vi "BuildConfigsFromFrontPanel.vi"(10 "AllControlsRefs":T25, 11 "InstruConfig":T1={"Mode"="", "InstrumentMode"={"MainDAQ_Selector"=enum."None", "LaserCtrlMethod"=enum."SRS_DG535", "InstruMode"=enum."fsLDPI"}, "CommuniationSettings"={"SDG_II"="", "DG535"="", "BNC565"="", "EPM2000"="", "NI-DAQmx"="", "Micos"={"Simulation"=FALSE, "ComPort"="", "Serial Config"={"Baud Rate"=0, "Parity"=0, "Data Bits"=0, "Stop Bits"=0, "Flow Control"=0}, "#Axis"=0}, "ESP300"={"Simulation"=FALSE, "ComPort"="", "Serial Config"={"Baud Rate"=0, "Parity"=0, "Data Bits"=0, "Stop Bits"=0, "Flow Control"=0}, "#Axis"=0}}, "DG535"={"Trigger"={"Trigger Mode"=enum."Internal", "Internal/Burst Rate"=0.0, "External  Level"=0.0, "Impedance"=FALSE, "Slope"=FALSE}, "Delays"=[], "Output"=[]}, "Gage_Config"={"Acquisition"={"Sample Rate"=0.0, "Mode"=0, "Start (0)"=0.0, "Depth"=0.0, "Segment Size"=0.0, "Trigger Delay"=0.0, "Trigger Timeout"=0.0, "Trigger Holdoff"=0.0, "Clock mode"=enum."Internal", "Segment"=1}, "Channels"=[], "Trigger"={"Slope"=0, "Level"=0, "Source"=0, "External Range"=0, "External Coupling"=0, "External"=FALSE, "Disable"=FALSE, "External Impedance"=0}, "Mode(Gage)"=enum."Normal"}, "AnalogDisc_Config"={"Acqusition"={"Freq(Hz,SampleRate)"=0.0, "BufferSize"=0, "Mode"=enum."Single", "RecordLength(s)"=0.0}, "Channels"=[], "Trigger"={"TriggerSource"=enum."None", "Timeout(s)"=0.0, "Holdoff(s)"=0.0, "Position/Delay(s)"=0.0}, "AnalogTrigger"={"Channel"=0, "Polarity"=enum."Rising", "Type"=enum."Edge", "Level(V)"=0.0, "Filter"=enum."Decimate", "Hysterisis(V)"=0.0}}, "Micos"={"Velocity"=0.0, "Acceleration"=0.0}, "ESP300"={"Velocity"=[], "Acceleration"=[]}, "EPM2000"={"Factor(A)"=0.0, "Factor(B)"=0.0}, "ProcessMethod"={"TopLine"=0.0, "Threshold"=0.0, "Baseline"=0.0, "ZeroOffset"=0.0, "Processing Mode"=enum."None"}, "Timing(LDPI)"={"Delay(PI)"=0.0, "Delay(Rejection)"=0.0, "NoDelayOffset"=0.0, "RepRate(Hz)"=0.0}, "Cali."=[0.0707, 0.16163, 0.02539], "BNC_Config"={"System"={"Rep.Rate"=1000.0, "Sys Ext Mode"=enum."Triggered", "Mode"=enum."Single Shot"}, "Channels"=[]}} {"Cali." format="%#.6f"; "Timing(LDPI)"."Delay(PI)" format="%#_6p"; "Timing(LDPI)"."Delay(Rejection)" format="%#_6p"; "Timing(LDPI)"."NoDelayOffset" format="%#_6p"; "DG535"."Trigger"."External  Level" min=-2.56 max=2.56 format="%.2f"; "DG535"."Trigger"."Internal/Burst Rate" min=0.001 max=1000000.0 format="%.3f"; "DG535"."Delays"."Delay" format="%#_6p"; "DG535"."Output"."Offset" min=-3.0 max=4.0 format="%.2f"; "DG535"."Output"."Amplitude" min=-3.0 max=4.0 format="%.2f"; "ProcessMethod"."Threshold" format="%#_6p"; "Gage_Config"."Trigger"."External Impedance" items=["50 Ohm", "HiZ"]; "Gage_Config"."Trigger"."External Coupling" items=["DC", "AC"]; "Gage_Config"."Trigger"."External Range" min=2000 max=10000 step=8000; "Gage_Config"."Trigger"."Slope" items=["Rising", "Falling"]; "Gage_Config"."Trigger"."Level" min=-100 max=100; "Gage_Config"."Trigger"."Source" min=0 max=64 step=1; "Gage_Config"."Channels"."Impedance" min=50 max=1000000 step=999950; "Gage_Config"."Channels"."Coupling" items=["DC", "AC"]; "Gage_Config"."Acquisition"."Segment Size" min=256.0 step=128.0; "Gage_Config"."Acquisition"."Trigger Delay" min=0.0 step=128.0; "Gage_Config"."Acquisition"."Trigger Timeout" format="%.0p"; "Gage_Config"."Acquisition"."Trigger Holdoff" min=0.0 step=128.0; "Gage_Config"."Acquisition"."Depth" min=256.0 step=128.0; "Gage_Config"."Acquisition"."Mode" items=["Single", "Dual", "Quad", "Octal"]; "Gage_Config"."Acquisition"."Sample Rate" format="%.0p"; "AnalogDisc_Config"."AnalogTrigger"."Level(V)" format="%#_6p"; "AnalogDisc_Config"."AnalogTrigger"."Hysterisis(V)" format="%#_6p"; "AnalogDisc_Config"."Acqusition"."RecordLength(s)" format="%#_6p"; "AnalogDisc_Config"."Acqusition"."Freq(Hz,SampleRate)" format="%#_6p"; "AnalogDisc_Config"."Trigger"."Position/Delay(s)" format="%#_6p"; "AnalogDisc_Config"."Trigger"."Holdoff(s)" format="%#_6p"; "AnalogDisc_Config"."Trigger"."Timeout(s)" format="%#_6p"}) -> (2 "InstruConfig out":T1={"Mode"="", "InstrumentMode"={"MainDAQ_Selector"=enum."None", "LaserCtrlMethod"=enum."SRS_DG535", "InstruMode"=enum."fsLDPI"}, "CommuniationSettings"={"SDG_II"="", "DG535"="", "BNC565"="", "EPM2000"="", "NI-DAQmx"="", "Micos"={"Simulation"=FALSE, "ComPort"="", "Serial Config"={"Baud Rate"=0, "Parity"=0, "Data Bits"=0, "Stop Bits"=0, "Flow Control"=0}, "#Axis"=0}, "ESP300"={"Simulation"=FALSE, "ComPort"="", "Serial Config"={"Baud Rate"=0, "Parity"=0, "Data Bits"=0, "Stop Bits"=0, "Flow Control"=0}, "#Axis"=0}}, "DG535"={"Trigger"={"Trigger Mode"=enum."Internal", "Internal/Burst Rate"=0.0, "External  Level"=0.0, "Impedance"=FALSE, "Slope"=FALSE}, "Delays"=[], "Output"=[]}, "Gage_Config"={"Acquisition"={"Sample Rate"=0.0, "Mode"=0, "Start (0)"=0.0, "Depth"=0.0, "Segment Size"=0.0, "Trigger Delay"=0.0, "Trigger Timeout"=0.0, "Trigger Holdoff"=0.0, "Clock mode"=enum."Internal", "Segment"=1}, "Channels"=[], "Trigger"={"Slope"=0, "Level"=0, "Source"=0, "External Range"=0, "External Coupling"=0, "External"=FALSE, "Disable"=FALSE, "External Impedance"=0}, "Mode(Gage)"=enum."Normal"}, "AnalogDisc_Config"={"Acqusition"={"Freq(Hz,SampleRate)"=0.0, "BufferSize"=0, "Mode"=enum."Single", "RecordLength(s)"=0.0}, "Channels"=[], "Trigger"={"TriggerSource"=enum."None", "Timeout(s)"=0.0, "Holdoff(s)"=0.0, "Position/Delay(s)"=0.0}, "AnalogTrigger"={"Channel"=0, "Polarity"=enum."Rising", "Type"=enum."Edge", "Level(V)"=0.0, "Filter"=enum."Decimate", "Hysterisis(V)"=0.0}}, "Micos"={"Velocity"=0.0, "Acceleration"=0.0}, "ESP300"={"Velocity"=[], "Acceleration"=[]}, "EPM2000"={"Factor(A)"=0.0, "Factor(B)"=0.0}, "ProcessMethod"={"TopLine"=0.0, "Threshold"=0.0, "Baseline"=0.0, "ZeroOffset"=0.0, "Processing Mode"=enum."None"}, "Timing(LDPI)"={"Delay(PI)"=0.0, "Delay(Rejection)"=0.0, "NoDelayOffset"=0.0, "RepRate(Hz)"=0.0}, "Cali."=[0.0707, 0.16163, 0.02539], "BNC_Config"={"System"={"Rep.Rate"=1000.0, "Sys Ext Mode"=enum."Triggered", "Mode"=enum."Single Shot"}, "Channels"=[]}} {"Cali." format="%#.6f"; "Timing(LDPI)"."Delay(PI)" format="%#_6p"; "Timing(LDPI)"."Delay(Rejection)" format="%#_6p"; "Timing(LDPI)"."NoDelayOffset" format="%#_6p"; "DG535"."Trigger"."External  Level" min=-2.56 max=2.56 format="%.2f"; "DG535"."Trigger"."Internal/Burst Rate" min=0.001 max=1000000.0 format="%.3f"; "DG535"."Delays"."Delay" format="%#_6p"; "DG535"."Output"."Offset" min=-3.0 max=4.0 format="%.2f"; "DG535"."Output"."Amplitude" min=-3.0 max=4.0 format="%.2f"; "ProcessMethod"."Threshold" format="%#_6p"; "Gage_Config"."Trigger"."External Impedance" items=["50 Ohm", "HiZ"]; "Gage_Config"."Trigger"."External Coupling" items=["DC", "AC"]; "Gage_Config"."Trigger"."External Range" min=2000 max=10000 step=8000; "Gage_Config"."Trigger"."Slope" items=["Rising", "Falling"]; "Gage_Config"."Trigger"."Level" min=-100 max=100; "Gage_Config"."Trigger"."Source" min=0 max=64 step=1; "Gage_Config"."Channels"."Impedance" min=50 max=1000000 step=999950; "Gage_Config"."Channels"."Coupling" items=["DC", "AC"]; "Gage_Config"."Acquisition"."Segment Size" min=256.0 step=128.0; "Gage_Config"."Acquisition"."Trigger Delay" min=0.0 step=128.0; "Gage_Config"."Acquisition"."Trigger Timeout" format="%.0p"; "Gage_Config"."Acquisition"."Trigger Holdoff" min=0.0 step=128.0; "Gage_Config"."Acquisition"."Depth" min=256.0 step=128.0; "Gage_Config"."Acquisition"."Mode" items=["Single", "Dual", "Quad", "Octal"]; "Gage_Config"."Acquisition"."Sample Rate" format="%.0p"; "AnalogDisc_Config"."AnalogTrigger"."Level(V)" format="%#_6p"; "AnalogDisc_Config"."AnalogTrigger"."Hysterisis(V)" format="%#_6p"; "AnalogDisc_Config"."Acqusition"."RecordLength(s)" format="%#_6p"; "AnalogDisc_Config"."Acqusition"."Freq(Hz,SampleRate)" format="%#_6p"; "AnalogDisc_Config"."Trigger"."Position/Delay(s)" format="%#_6p"; "AnalogDisc_Config"."Trigger"."Holdoff(s)" format="%#_6p"; "AnalogDisc_Config"."Trigger"."Timeout(s)" format="%#_6p"})   [LabVIEW 2013]
uses:
  ControlDef/InstrumentConfiguration.ctl
  ControlDef/MainDAQ_Selector.ctl
  ControlDef/LaserCtrl_Method.ctl
  ControlDef/InstruMode_Typedef.ctl
  <instrlib>/DG535/Command/Set Trigger.ctl
  <instrlib>/DG535/Command/DG535_TriggerMode.ctl
  <instrlib>/DG535/Command/Set Delay.ctl
  <instrlib>/DG535/Command/DG535_Channel.ctl
  <instrlib>/DG535/Command/Set Output.ctl
  <instrlib>/DG535/Command/DG535_Output.ctl
  <instrlib>/GageLv_uic/VI/Gage_Configs.ctl
  <instrlib>/AnalogDiscSDKLv/VIs/DWF_AnalogIn_Configurations.ctl
  <instrlib>/AnalogDiscSDKLv/VIs/DWF_AcqMode.ctl
  <instrlib>/AnalogDiscSDKLv/VIs/DWF_Filter.ctl
  <instrlib>/AnalogDiscSDKLv/VIs/DWF_TrigSrc.ctl
  <instrlib>/AnalogDiscSDKLv/VIs/DWF_TrigCond.ctl
  <instrlib>/AnalogDiscSDKLv/VIs/DWF_TrigType.ctl
  ControlDef/ProcessingMode.ctl
  Hardware/BNC(QuantumComposers)/BNC_Configs.ctl
  ControlDef/InstrumentSpecificControls/UIC-AToF/InitializationParams_BNC565_2Ch_AToF.ctl
  Hardware/BNC(QuantumComposers)/Command/Set C-Input.ctl
  Hardware/BNC(QuantumComposers)/Command/Set C-Mode.ctl
  Hardware/BNC(QuantumComposers)/Command/Set C-Output.ctl
  Hardware/BNC(QuantumComposers)/Command/Set C-Enable.ctl
  ControlDef/AllControlsRefs.ctl
  <instrlib>/DG535/SRS_DG535_Lib.lvlib
  <instrlib>/GageLv_uic/Gage.lvlib
  <instrlib>/AnalogDiscSDKLv/AnalogDiscSDKLv.lvlib
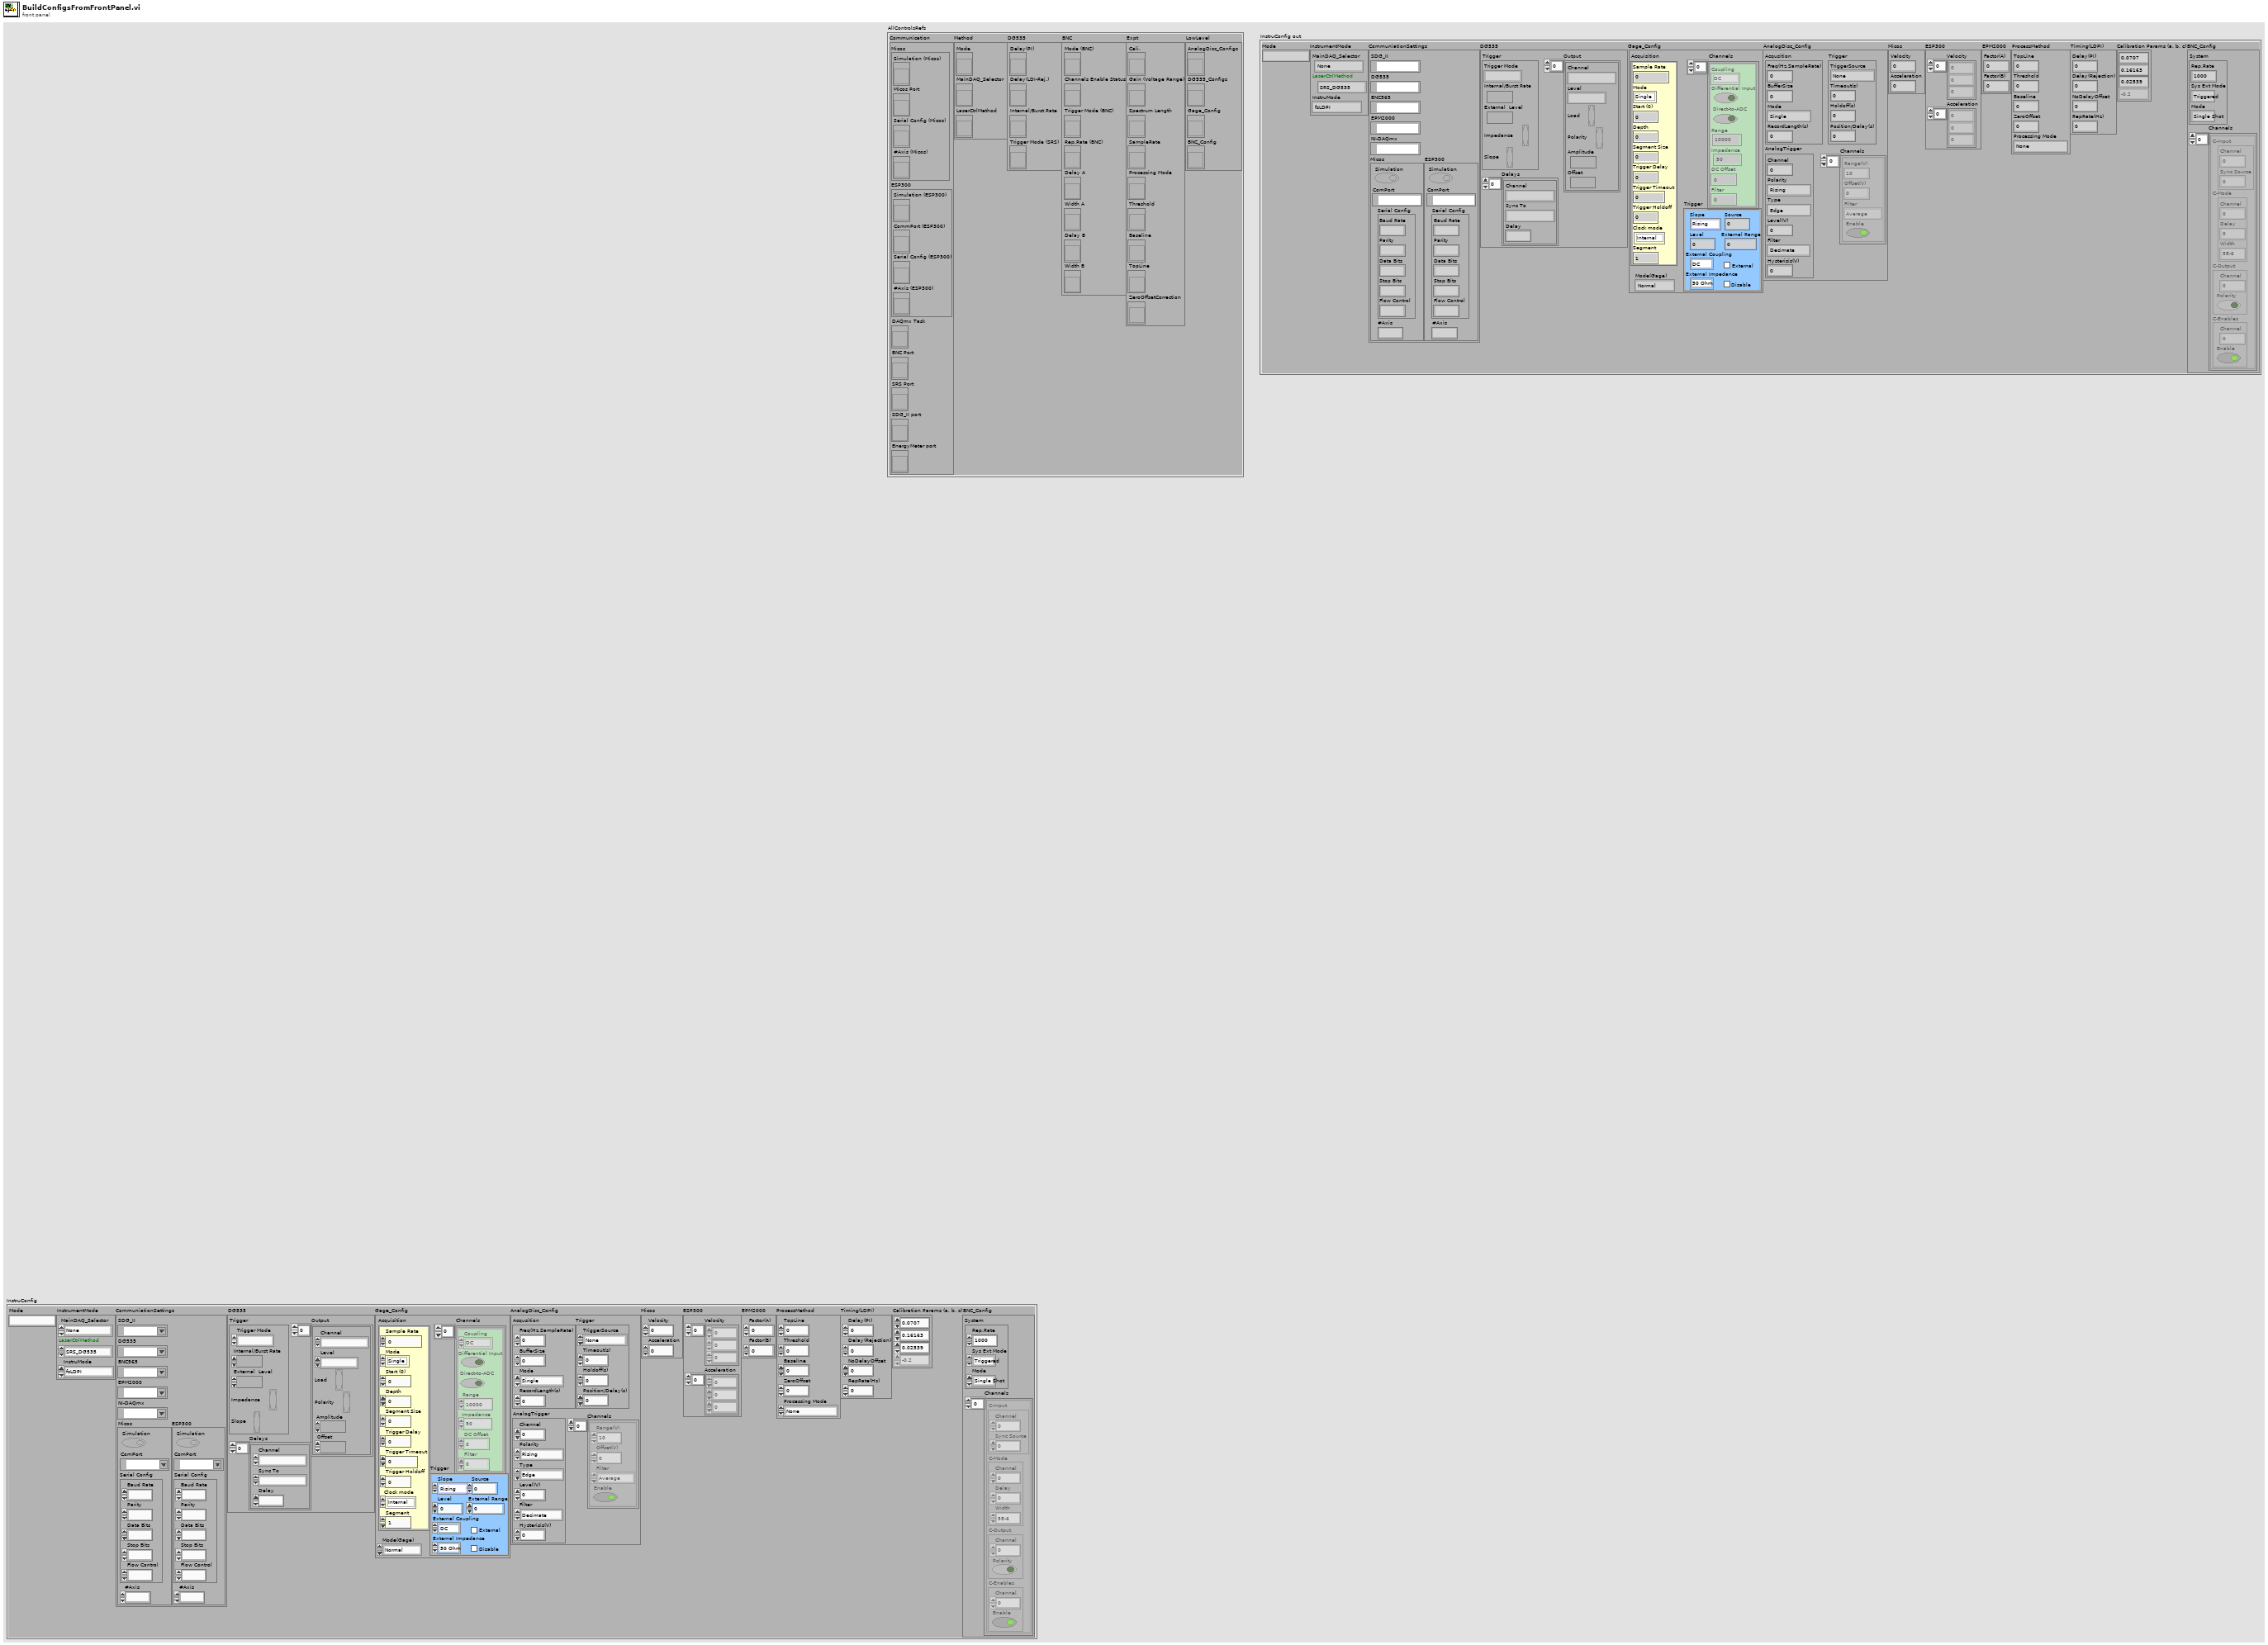
[diagram p1: front panel]
types:
  T1 = typedef "InstrumentConfiguration.ctl" = cluster{"Mode":string, "InstrumentMode":cluster{"MainDAQ_Selector":T2, "LaserCtrlMethod":T3, "InstruMode":T4}, "CommuniationSettings":cluster{"SDG_II":refnum<visa-resource-name>, "DG535":refnum<visa-resource-name>, "BNC565":refnum<visa-resource-name>, "EPM2000":refnum<visa-resource-name>, "NI-DAQmx":refnum<visa-resource-name>, "Micos":cluster{"Simulation":bool, "ComPort":refnum<visa-resource-name>, "Serial Config":cluster{"Baud Rate":u32, "Parity":u16, "Data Bits":u16, "Stop Bits":u16, "Flow Control":u16}, "#Axis":i32}, "ESP300":cluster{"Simulation":bool, "ComPort":refnum<visa-resource-name>, "Serial Config":cluster{"Baud Rate":u32, "Parity":u16, "Data Bits":u16, "Stop Bits":u16, "Flow Control":u16}, "#Axis":i32}}, "DG535":cluster{"Trigger":T5, "Delays":T7[], "Output":T9[]}, "Gage_Config":T11, "AnalogDisc_Config":T12, "Micos":cluster{"Velocity":dbl, "Acceleration":dbl}, "ESP300":cluster{"Velocity":dbl[], "Acceleration":dbl[]}, "EPM2000":cluster{"Factor(A)":dbl, "Factor(B)":dbl}, "ProcessMethod":cluster{"TopLine":dbl, "Threshold":dbl, "Baseline":dbl, "ZeroOffset":dbl, "Processing Mode":T18}, "Timing(LDPI)":cluster{"Delay(PI)":dbl, "Delay(Rejection)":dbl, "NoDelayOffset":dbl, "RepRate(Hz)":dbl}, "Cali.":dbl[], "BNC_Config":T19}
  T2 = typedef "MainDAQ_Selector.ctl" = enum16{"None", "Gage", "Gage_AdvMultiRec_8bit1Ch", "IonWerks_TDCx4", "Tektronics", "KnifeEdge_Emu", "AnalogDisc", "Gage_AMR_8bit2Ch", "Gage_AMR_16bit1Ch", "Gage_AMR_16bit2Ch"}
  T3 = typedef "LaserCtrl_Method.ctl" = enum16{"SRS_DG535", "BNC", "SDG_II"}
  T4 = typedef "InstruMode_Typedef.ctl" = enum16{"fsLDPI", "nsLDPI", "nsLD-fsPI", "GenericTOF", "BeamProfiling"}
  T5 = typedef "SRS_DG535_Lib.lvlib/Set Trigger.ctl" = cluster{"Trigger Mode":T6, "Internal/Burst Rate":dbl, "External  Level":sgl, "Impedance":bool, "Slope":bool}
  T6 = typedef "SRS_DG535_Lib.lvlib/DG535_TriggerMode.ctl" = enum16{"Internal", "External", "SingleShot", "Burst", "Line"}
  T7 = typedef "SRS_DG535_Lib.lvlib/Set Delay.ctl" = cluster{"Channel":T8, "Sync To":T8, "Delay":dbl}
  T8 = typedef "SRS_DG535_Lib.lvlib/DG535_Channel.ctl" = enum16{"Trigger Input", "T0 Output", "A Output", "B Output", "AB Output", "C Output", "D Output", "CD Output", "NULL"}
  T9 = typedef "SRS_DG535_Lib.lvlib/Set Output.ctl" = cluster{"Channel":T8, "Level":T10, "Load":bool, "Polarity":bool, "Amplitude":dbl, "Offset":dbl}
  T10 = typedef "SRS_DG535_Lib.lvlib/DG535_Output.ctl" = enum16{"TTL", "NIM", "ECL", "Variable"}
  T11 = typedef "Gage.lvlib/Gage_Configs.ctl" = cluster{"Acquisition":cluster{"Sample Rate":dbl, "Mode":u16, "Start (0)":dbl, "Depth":dbl, "Segment Size":dbl, "Trigger Delay":dbl, "Trigger Timeout":dbl, "Trigger Holdoff":dbl, "Clock mode":enum16{"Internal", "External", "Reference"}, "Segment":u32}, "Channels":cluster{"Coupling":u16, "Differential Input":bool, "Direct-to-ADC":bool, "Range":u32, "Impedance":u32, "DC Offset":i32, "Filter":i32}[], "Trigger":cluster{"Slope":u16, "Level":i32, "Source":i32, "External Range":u32, "External Coupling":u16, "External":bool, "Disable":bool, "External Impedance":u16}, "Mode(Gage)":enum16{"Normal", "Continuous", "MultiRecord", "HwAverage"}}
  T12 = typedef "AnalogDiscSDKLv.lvlib/DWF_AnalogIn_Configurations.ctl" = cluster{"Acqusition":cluster{"Freq(Hz,SampleRate)":dbl, "BufferSize":i32, "Mode":T13, "RecordLength(s)":dbl}, "Channels":cluster{"Range(V)":dbl, "Offset(V)":dbl, "Filter":T14, "Enable":bool}[], "Trigger":cluster{"TriggerSource":T15, "Timeout(s)":dbl, "Holdoff(s)":dbl, "Position/Delay(s)":dbl}, "AnalogTrigger":cluster{"Channel":i32, "Polarity":T16, "Type":T17, "Level(V)":dbl, "Filter":T14, "Hysterisis(V)":dbl}}
  T13 = typedef "AnalogDiscSDKLv.lvlib/DWF_AcqMode.ctl" = enum16{"Single", "ScanShift", "ScanScreen", "Record"}
  T14 = typedef "AnalogDiscSDKLv.lvlib/DWF_Filter.ctl" = enum16{"Decimate", "Average", "MinMax"}
  T15 = typedef "AnalogDiscSDKLv.lvlib/DWF_TrigSrc.ctl" = enum16{"None", "PC", "DetectorAnalogIn", "DetectorDigitalIn", "AnalogIn", "DigitalIn", "DigitalOut", "AnalogOut1", "AnalogOut2", "AnalogOut3", "AnalogOut4", "External1", "External2", "External3", "External4"}
  T16 = typedef "AnalogDiscSDKLv.lvlib/DWF_TrigCond.ctl" = enum16{"Rising", "Falling"}
  T17 = typedef "AnalogDiscSDKLv.lvlib/DWF_TrigType.ctl" = enum16{"Edge", "Pulse", "Transition"}
  T18 = typedef "ProcessingMode.ctl" = enum16{"None", "Drop by Threshold", "TDC Simulate", "SetFilter"}
  T19 = typedef "BNC_Configs.ctl" = cluster{"System":cluster{"Rep.Rate":dbl, "Sys Ext Mode":enum16{"Disabled", "Triggered", "Gated", "Triggered & Gated"}, "Mode":enum16{"Normal", "Single Shot", "Duty Cycle", "Burst"}}, "Channels":T20[]}
  T20 = typedef "InitializationParams_BNC565_2Ch_AToF.ctl" = cluster{"C-Input":T21, "C-Mode":T22, "C-Output":T23, "C-Enables":T24}
  T21 = typedef "Set C-Input.ctl" = cluster{"Channel":i32, "Sync Source":i32}
  T22 = typedef "Set C-Mode.ctl" = cluster{"Channel":i32, "Delay":dbl, "Width":dbl}
  T23 = typedef "Set C-Output.ctl" = cluster{"Channel":i32, "Polarity":bool}
  T24 = typedef "Set C-Enable.ctl" = cluster{"Channel":i32, "Enable":bool}
  T25 = typedef "AllControlsRefs.ctl" = cluster{"Communication":cluster{"Micos":cluster{"Simulation (Micos)":refnum<vi>, "Micos Port":refnum<vi>, "Serial Config (Micos)":refnum<vi>, "#Axis (Micos)":refnum<vi>}, "ESP300":cluster{"Simulation (ESP300)":refnum<vi>, "CommPort (ESP300)":refnum<vi>, "Serial Config (ESP300)":refnum<vi>, "#Axis (ESP300)":refnum<vi>}, "DAQmx Task":refnum<vi>, "BNC Port":refnum<vi>, "SRS Port":refnum<vi>, "SDG_II port":refnum<vi>, "EnergyMeter port":refnum<vi>}, "Method":cluster{"Mode":refnum<vi>, "MainDAQ_Selector":refnum<vi>, "LaserCtrlMethod":refnum<vi>}, "DG535":cluster{"Delay(PI)":refnum<vi>, "Delay(LDI-Rej.)":refnum<vi>, "Internal/Burst Rate":refnum<vi>, "Trigger Mode (SRS)":refnum<vi>}, "BNC":cluster{"Mode (BNC)":refnum<vi>, "Channels Enable Status":refnum<vi>, "Trigger Mode (BNC)":refnum<vi>, "Rep.Rate (BNC)":refnum<vi>, "Delay A":refnum<vi>, "Width A":refnum<vi>, "Delay B":refnum<vi>, "Width B":refnum<vi>}, "Expt":cluster{"Cali.":refnum<vi>, "Gain (Voltage Range)":refnum<vi>, "Spectrum Length":refnum<vi>, "SampleRate":refnum<vi>, "Processing Mode":refnum<vi>, "Threshold":refnum<vi>, "Baseline":refnum<vi>, "TopLine":refnum<vi>, "ZeroOffsetCorrection":refnum<vi>}, "LowLevel":cluster{"AnalogDisc_Configs":refnum<vi>, "DG535_Configs":refnum<vi>, "Gage_Config":refnum<vi>, "BNC_Config":refnum<vi>}}
  T26 = cluster{"Trigger":T5, "Delays":T7[], "Output":T9[]}
  T27 = cluster{"Baud Rate":u32, "Parity":u16, "Data Bits":u16, "Stop Bits":u16, "Flow Control":u16}
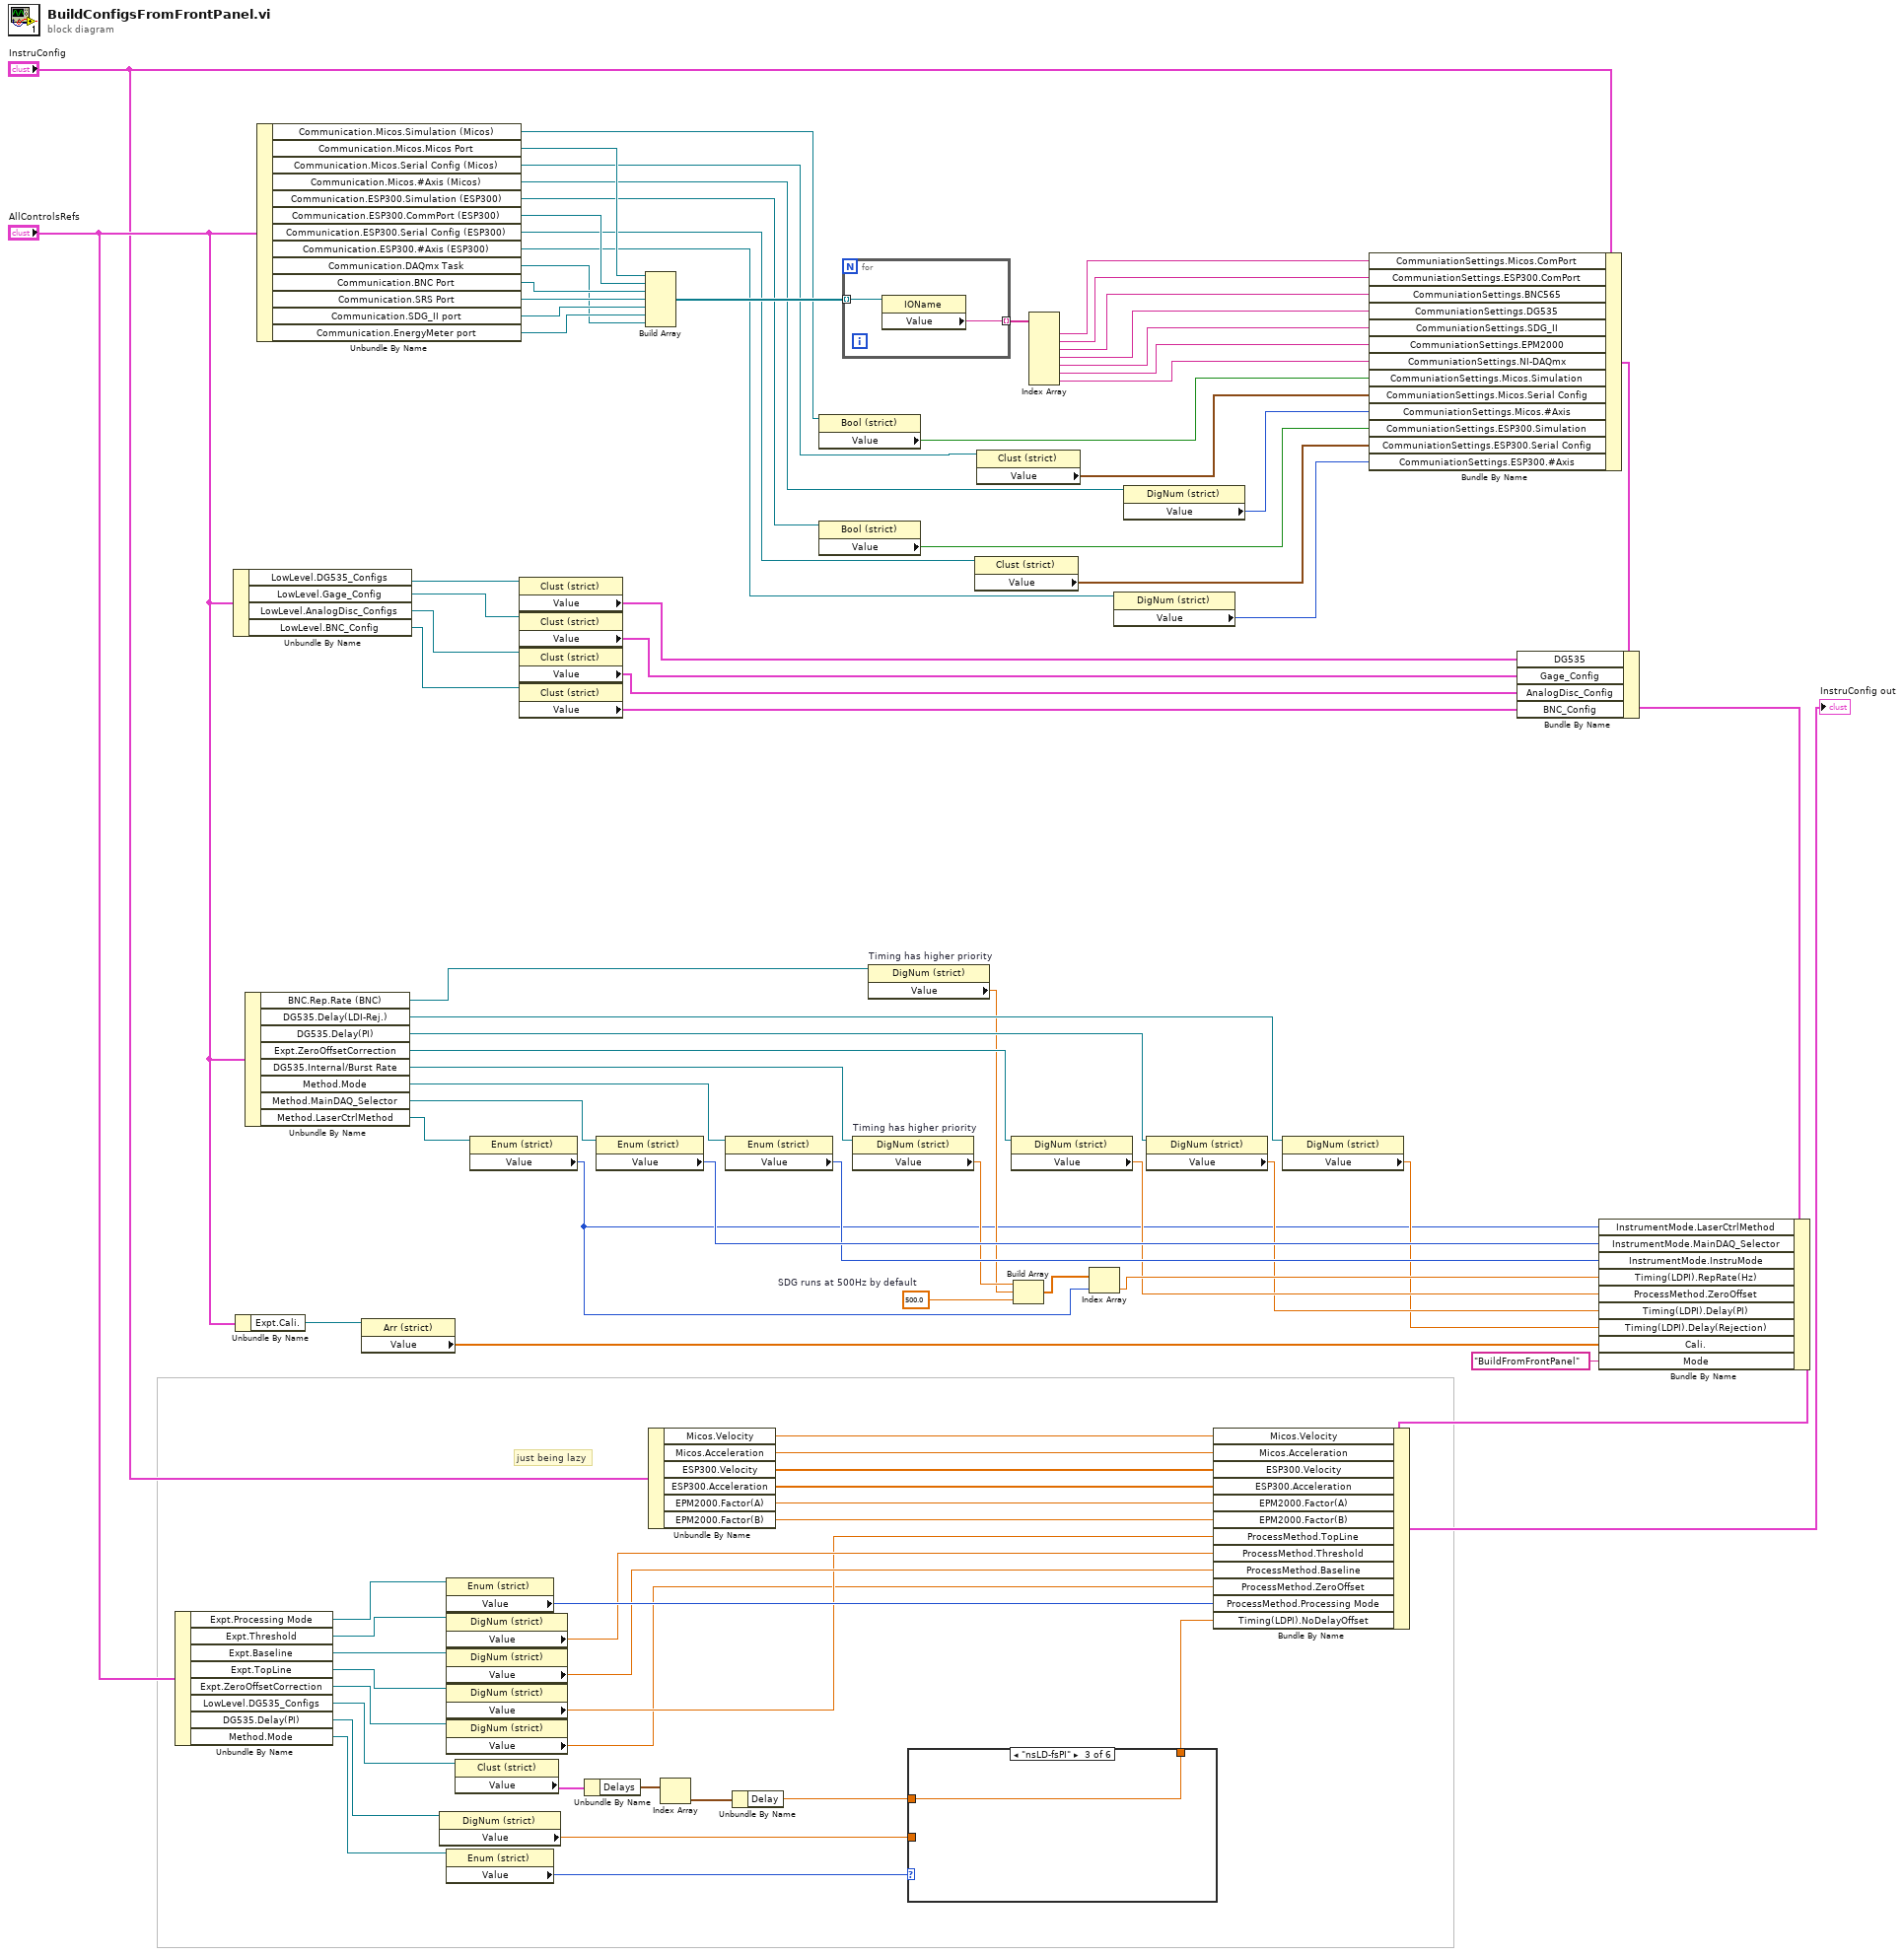
[diagram p0: block diagram]
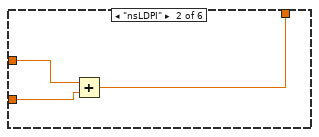
[diagram p3: hidden frame]
diagram:
  w34 = 500.0  # SDG runs at 500Hz by default
  # "just being lazy"
  n1 = Unbundle By Name("AllControlsRefs") -> ("Expt.Processing Mode"=w28:refnum<vi>, "Expt.Threshold"=w27:refnum<vi>, "Expt.Baseline"=w26:refnum<vi>, "Expt.TopLine"=w25:refnum<vi>, "Expt.ZeroOffsetCorrection"=w24:refnum<vi>, "LowLevel.DG535_Configs"=w10:refnum<vi>, "DG535.Delay(PI)"=w2:refnum<vi>, "Method.Mode"=w6:refnum<vi>)
  n2 = Unbundle By Name("AllControlsRefs") -> ("LowLevel.DG535_Configs"=w83:refnum<vi>, "LowLevel.Gage_Config"=w82:refnum<vi>, "LowLevel.AnalogDisc_Configs"=w81:refnum<vi>, "LowLevel.BNC_Config"=w65:refnum<vi>)
  n3 = Unbundle By Name("AllControlsRefs") -> ("Expt.Cali."=w66:refnum<vi>)
  n4 = Unbundle By Name("AllControlsRefs") -> ("BNC.Rep.Rate (BNC)"=w35:refnum<vi>, "DG535.Delay(LDI-Rej.)"=w67:refnum<vi>, "DG535.Delay(PI)"=w68:refnum<vi>, "Expt.ZeroOffsetCorrection"=w69:refnum<vi>, "DG535.Internal/Burst Rate"=w70:refnum<vi>, "Method.Mode"=w73:refnum<vi>, "Method.MainDAQ_Selector"=w72:refnum<vi>, "Method.LaserCtrlMethod"=w71:refnum<vi>)
  n5 = Unbundle By Name("AllControlsRefs") -> ("Communication.Micos.Simulation (Micos)"=w80:refnum<vi>, "Communication.Micos.Micos Port"=w90:refnum<vi>, "Communication.Micos.Serial Config (Micos)"=w78:refnum<vi>, "Communication.Micos.#Axis (Micos)"=w77:refnum<vi>, "Communication.ESP300.Simulation (ESP300)"=w79:refnum<vi>, "Communication.ESP300.CommPort (ESP300)"=w89:refnum<vi>, "Communication.ESP300.Serial Config (ESP300)"=w76:refnum<vi>, "Communication.ESP300.#Axis (ESP300)"=w75:refnum<vi>, "Communication.DAQmx Task"=w74:refnum<vi>, "Communication.BNC Port"=w88:refnum<vi>, "Communication.SRS Port"=w87:refnum<vi>, "Communication.SDG_II port"=w86:refnum<vi>, "Communication.EnergyMeter port"=w85:refnum<vi>)
  n6 = property class="Arr (strict)"(reference=w66) -> ("Value"=w42:dbl[])  [unwired: 1 in, 2 out]
  n7 = property class="DigNum (strict)"(reference=w2) -> ("Value"=w1:dbl)  [unwired: 1 in, 2 out]
  n8 = property class="Enum (strict)"(reference=w28) -> ("Value"=w23:T18)  [unwired: 1 in, 2 out]
  n9 = property class="DigNum (strict)"(reference=w27) -> ("Value"=w22:dbl)  [unwired: 1 in, 2 out]
  n10 = property class="DigNum (strict)"(reference=w26) -> ("Value"=w21:dbl)  [unwired: 1 in, 2 out]
  n11 = property class="DigNum (strict)"(reference=w25) -> ("Value"=w20:dbl)  [unwired: 1 in, 2 out]
  n12 = property class="DigNum (strict)"(reference=w24) -> ("Value"=w19:dbl)  [unwired: 1 in, 2 out]
  n13 = property class="Enum (strict)"(reference=w6) -> ("Value"=w5:T4)  [unwired: 1 in, 2 out]
  n14 = property class="Clust (strict)"(reference=w10) -> ("Value"=w9:T26)  [unwired: 1 in, 2 out]
  n15 = property class="Enum (strict)"(reference=w71) -> ("Value"=w30:T3)  [unwired: 1 in, 2 out]
  n16 = property class="Clust (strict)"(reference=w83) -> ("Value"=w62:T26)  [unwired: 1 in, 2 out]
  n17 = property class="Clust (strict)"(reference=w82) -> ("Value"=w61:T11)  [unwired: 1 in, 2 out]
  n18 = property class="Clust (strict)"(reference=w81) -> ("Value"=w60:T12)  [unwired: 1 in, 2 out]
  n19 = property class="Clust (strict)"(reference=w65) -> ("Value"=w59:T19)  [unwired: 1 in, 2 out]
  n20 = Unbundle By Name(w9) -> ("Delays"=w8:T7[])
  n21 = property class="Enum (strict)"(reference=w72) -> ("Value"=w41:T2)  [unwired: 1 in, 2 out]
  n22 = Build Array(w90, w89, w88, w87, w86, w85, w74) -> (w84:refnum<vi>[])
  n23 = Unbundle By Name("InstruConfig") -> ("Micos.Velocity"=w17:dbl, "Micos.Acceleration"=w16:dbl, "ESP300.Velocity"=w15:dbl[], "ESP300.Acceleration"=w14:dbl[], "EPM2000.Factor(A)"=w13:dbl, "EPM2000.Factor(B)"=w12:dbl)
  n24 = Index Array(array=w8) -> (element=w7:T7)  [unwired: 1 in]
  n25 = property class="Enum (strict)"(reference=w73) -> ("Value"=w40:T4)  [unwired: 1 in, 2 out]
  n26 = Unbundle By Name(w7) -> ("Delay"=w3:dbl)
  n27 = property class="Bool (strict)"(reference=w80) -> ("Value"=w49:bool)  [unwired: 1 in, 2 out]
  n28 = property class="Bool (strict)"(reference=w79) -> ("Value"=w46:bool)  [unwired: 1 in, 2 out]
  n29 = for {
    tunnel: w84 -> [w92] mode=indexing
    tunnel: [w91] -> w57 mode=indexing
    n30 = property class="IOName"(reference=w92) -> ("Value"=w91:string)  [unwired: 1 in, 2 out]
  }
  n31 = property on="Timing has higher priority" class="DigNum (strict)"(reference=w70) -> ("Value"=w33:dbl)  [unwired: 1 in, 2 out]
  n32 = property on="Timing has higher priority" class="DigNum (strict)"(reference=w35) -> ("Value"=w32:dbl)  [unwired: 1 in, 2 out]
  n33 = case shown="\"nsLD-fsPI\"" w5 {
    tunnel: [w93 w94 w97 _ _ _] -> w4
    tunnel: w3 -> [w93 w95 w97 _ _ _]
    tunnel: w1 -> [_ w96 _ _ _ _]
    frame "fsLDPI" {
    }
    frame "nsLDPI" {
      n34 = Add(x=w95, y=w96) -> (x+y=w94:dbl)
    }
    frame "nsLD-fsPI" {
    }
    frame "GenericTOF" {
    }
    frame Default {
    }
    frame "BeamProfiling" {
    }
  }
  n35 = property class="Clust (strict)"(reference=w76) -> ("Value"=w45:T27)  [unwired: 1 in, 2 out]
  n36 = property class="Clust (strict)"(reference=w78) -> ("Value"=w48:T27)  [unwired: 1 in, 2 out]
  n37 = property class="DigNum (strict)"(reference=w69) -> ("Value"=w38:dbl)  [unwired: 1 in, 2 out]
  n38 = Build Array(w33, w32, w34) -> (w31:dbl[])
  n39 = Index Array(array=w57) -> (element #1=w56:string, element #2=w54:string, element #3=w55:string, element #4=w53:string, element #5=w52:string, element #6=w51:string, element #7=w50:string)  [unwired: 7 in]
  n40 = Index Array(array=w31, index=w30) -> (element=w39:dbl)
  n41 = property class="DigNum (strict)"(reference=w75) -> ("Value"=w44:i32)  [unwired: 1 in, 2 out]
  n42 = property class="DigNum (strict)"(reference=w77) -> ("Value"=w47:i32)  [unwired: 1 in, 2 out]
  n43 = property class="DigNum (strict)"(reference=w68) -> ("Value"=w37:dbl)  [unwired: 1 in, 2 out]
  n44 = property class="DigNum (strict)"(reference=w67) -> ("Value"=w36:dbl)  [unwired: 1 in, 2 out]
  n45 = Bundle By Name(cluster="InstruConfig", "CommuniationSettings.Micos.ComPort"=w56, "CommuniationSettings.ESP300.ComPort"=w54, "CommuniationSettings.BNC565"=w55, "CommuniationSettings.DG535"=w53, "CommuniationSettings.SDG_II"=w52, "CommuniationSettings.EPM2000"=w51, "CommuniationSettings.NI-DAQmx"=w50, "CommuniationSettings.Micos.Simulation"=w49, "CommuniationSettings.Micos.Serial Config"=w48, "CommuniationSettings.Micos.#Axis"=w47, "CommuniationSettings.ESP300.Simulation"=w46, "CommuniationSettings.ESP300.Serial Config"=w45, "CommuniationSettings.ESP300.#Axis"=w44) -> (w58:T1)
  n46 = Bundle By Name(cluster=w58, "DG535"=w62, "Gage_Config"=w61, "AnalogDisc_Config"=w60, "BNC_Config"=w59) -> (w63:T1)
  n47 = Bundle By Name(cluster=w63, "InstrumentMode.LaserCtrlMethod"=w30, "InstrumentMode.MainDAQ_Selector"=w41, "InstrumentMode.InstruMode"=w40, "Timing(LDPI).RepRate(Hz)"=w39, "ProcessMethod.ZeroOffset"=w38, "Timing(LDPI).Delay(PI)"=w37, "Timing(LDPI).Delay(Rejection)"=w36, "Cali."=w42, "Mode"="BuildFromFrontPanel") -> (w43:T1)
  n48 = Bundle By Name(cluster=w43, "Micos.Velocity"=w17, "Micos.Acceleration"=w16, "ESP300.Velocity"=w15, "ESP300.Acceleration"=w14, "EPM2000.Factor(A)"=w13, "EPM2000.Factor(B)"=w12, "ProcessMethod.TopLine"=w20, "ProcessMethod.Threshold"=w22, "ProcessMethod.Baseline"=w21, "ProcessMethod.ZeroOffset"=w19, "ProcessMethod.Processing Mode"=w23, "Timing(LDPI).NoDelayOffset"=w4) -> (→"InstruConfig out":T1)
